vi "Read s4 acq config errors.vi"(8 "error in (no error)":errorcluster, 11 "SPARC4_Channel in":refnum<class "SPARC4_Channel.lvclass">) -> (0 "error out":errorcluster, 1 "acquisition config errors":T1, 2 "s4 acq config errors":T2, 3 "SPARC4_Channel out":refnum<class "SPARC4_Channel.lvclass">)   [LabVIEW 2018, in "SPARC4_Channel.lvclass"]
uses:
  SPARC4_Channel.lvclass
  SPARC4_Channel.lvclass/SPARC4_Channel.ctl
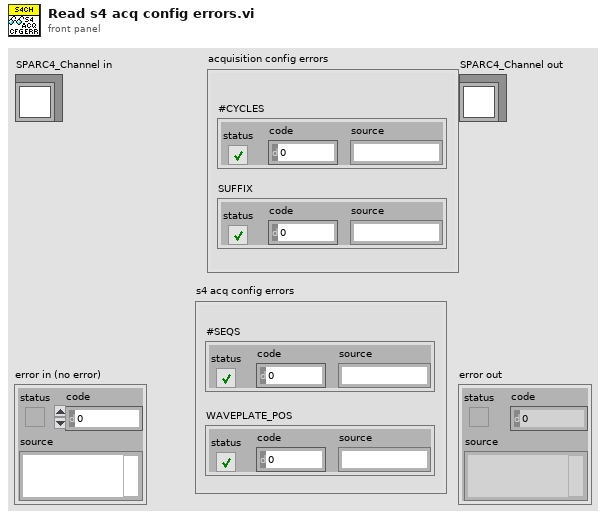
[diagram p1: front panel]
types:
  T1 = cluster{"#CYCLES":errorcluster, "SUFFIX":errorcluster}
  T2 = cluster{"#SEQS":errorcluster, "WAVEPLATE_POS":errorcluster}
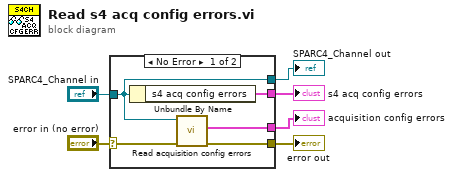
[diagram p0: block diagram]
diagram:
  n1 = case shown="No Error" "error in (no error)" {
    selector: "error in (no error)" -> [w10 w12]
    tunnel: [w8 w12] -> w5
    tunnel: [w9 w13] -> w3
    tunnel: "SPARC4_Channel in" -> [w9 w13]
    tunnel: [w11 _] -> w2
    tunnel: [w7 _] -> w1
    frame No Error {
      n2 = Unbundle By Name(w9) -> ("s4 acq config errors"=w11:T2)
      n3 = call-dynamic "Read acquisition config errors.vi"("error in (no error)"=w10, "Channel in"=w9) -> ("error out"=w8:errorcluster, "acquisition config errors"=w7:T1)  [unwired: 7 in, 1 out]
    }
    frame Error {
    }
  }
  "error out" <- w5
  "SPARC4_Channel out" <- w3
  "s4 acq config errors" <- w2
  "acquisition config errors" <- w1
